vi "COMI DO Put All Ex.vi"(9 "dwStatuses":u32, 10 "nGroupIdx":i32, 11 "hDevice":u32) -> (3 "hDevice out":u32)   [LabVIEW 2017, in "Comidll.lvlib"]
doc: "void (COMI_DO_PutAllEx) (HANDLE hDevice, int nGroupIdx, unsigned long dwStatuses);"
uses:
  <userlib>/Comidll/Comidll.lvlib
  <userlib>/Comidll/Comidll.dll
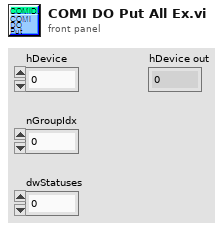
[diagram p1: front panel]
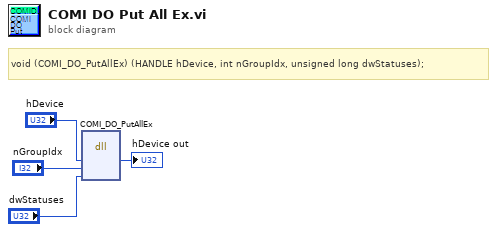
[diagram p0: block diagram]
diagram:
  # "void\t(COMI_DO_PutAllEx) (HANDLE hDevice, int nGroupIdx, unsigned long dwStatuses);"
  n1 = dll-call lib="C:/Program Files/National Instruments/LabVIEW 2017/user.lib/Comidll/Comidll.*" fn="COMI_DO_PutAllEx"("hDevice"="hDevice", "nGroupIdx"="nGroupIdx", "dwStatuses"="dwStatuses") -> ("hDevice"=→"hDevice out":u32)  [unwired: 6 in, 2 out]
